vi "Matrix To Array.vi"   [LabVIEW 2010, in "NI_Matrix.lvlib"]
doc: "Converts a matrix of elements to an array of elements of the same data type. Wire data to the <B>Real Matrix</B> input to determine the polymorphic instance to use or manually select the instance."
uses:
  NI_Matrix.lvlib
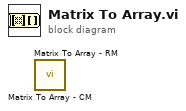
[diagram p0: block diagram]
diagram:
  n1 = call "Matrix To Array - CM.vi"() -> ()  [unwired: 1 in, 1 out]
  n2 = call "Matrix To Array - RM.vi"() -> ()  [unwired: 1 in, 1 out]
